vi "Basic Serial Write and Read_COM.vi"(0 "Setting":T1={"VISA resource name"="COM1", "baud rate"=57600, "data bits"=8, "parity"=0, "stop bits"=10, "flow control"=0, "Read TimeOut (ms)"=500, "Byte Read Count(999Exit)"=500, "Read End Str"=FALSE, "End String"=""} {"flow control" items=["None"=0, "XON/XOFF"=1, "RTS/CTS"=2, "DTR/DSR"=4]; "stop bits" items=["1.0"=10, "1.5"=15, "2.0"=20]; "parity" items=["None", "Odd", "Even", "Mark", "Space"]; "data bits" min=5 max=8 step=1}, 2 "string to write":string="*IDN?\n", 3 "Open":bool, 5 "write":bool=TRUE, 6 "read":bool=TRUE) -> (9 "read string":string, 10 "bytes read":u32)   [LabVIEW 2016]
doc: "The Basic Serial Read and Write example performs a Serial Port Read, a Serial Port Write, or a combination of these actions. The user selects the actions (read or write) on the front panel. If both are selected, the VI will write the data first, read data, and then close the VISA session that is opened to the port. This VI will wait until the specified number of bytes is received at the port or until a termination character is read.\n\nINSTRUCTIONS:\n1) Select the serial resource and configuration parameters (baud rate, data bits, parity, stop bits, flow control).\n2) Select the operations to be performed. \n3) Connect the serial port to your device. If no device is available, perform a loopback test by doing one of the following. Short pins 2 and 3 on a RS-232 cable or short pin 4 to pin 8 and pin 5 to pin 9 on a RS-485/422 cable. \n4) Run the VI to see the data read. (The \"read string\" will match the \"string to write\" if a loopback test was performed.)\n\nNote: The parameters set for the serial port must match the parameters of the connected instrument or device. In this example, the bytes to read parameter specifies the number of bytes that the serial port reads. If there were more bytes at the port than the number specified in bytes to read, those bytes would not be read. Also, if you specify to read more bytes than the number of bytes actually read, you might receive a timeout error message.\n\nOn the block diagram, the Configure Serial Port VI sets the configuration parameters. The front panel displays the controls used to configure the basic parameters, such as baud rate, data bits, and parity. Constants configure the other parameters the user probably does not need set. After the VISA Configure Serial Port VI opens the VISA session and configures the port, the VI passes the VISA resource name to other VIs that perform operations on that VISA resource. The VISA Write function sends a command to the serial device and the VISA Read function returns data based on the command. The VISA Close function then closes the reference to the serial device. It is important to close the reference; otherwise communication through with that port through protocols other than VISA might not be possible."
uses:
  <vilib>/Instr/_visa.llb/VISA Configure Serial Port (Instr).vi
panel:
  out "read buffer":string
  out "Tact Time":u32
  out "return count":u32
  # "On Windows/Linux, consider using the Instrument Driver Finder (Help>>Find Instrument Drivers) to search for an instrument driver for your instrument."
  # "Select the serial resource and the operations (Read, Write, or both) to be performed.  If both are selected, the VI will write the data first, read data and then close the VISA session that is opened to the port.  This VI will wait until the specified number of bytes is received at the port or until a termination character is read."
  # "For additional information select File >> VI Properties >> Documentation"
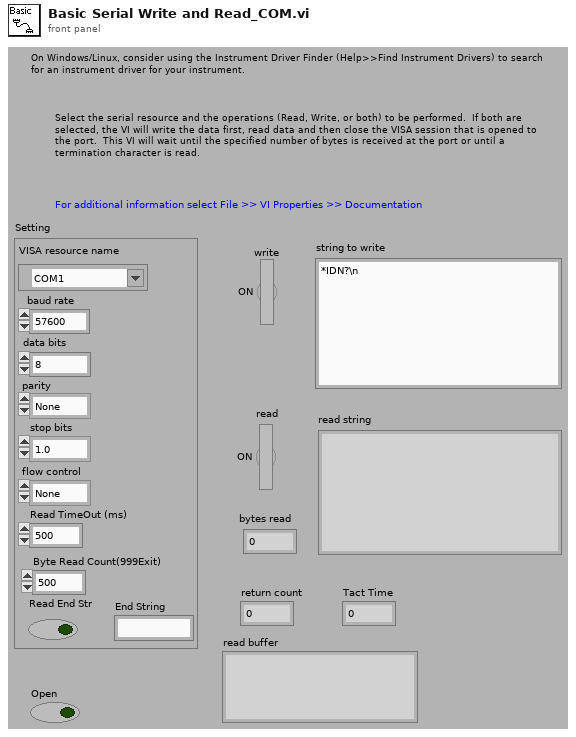
[diagram p1: front panel]
types:
  T1 = cluster{"VISA resource name":refnum<visa-resource-name>, "baud rate":u32, "data bits":u16, "parity":u16, "stop bits":u16, "flow control":u16, "Read TimeOut (ms)":u32, "Byte Read Count(999Exit)":u32, "Read End Str":bool, "End String":string}
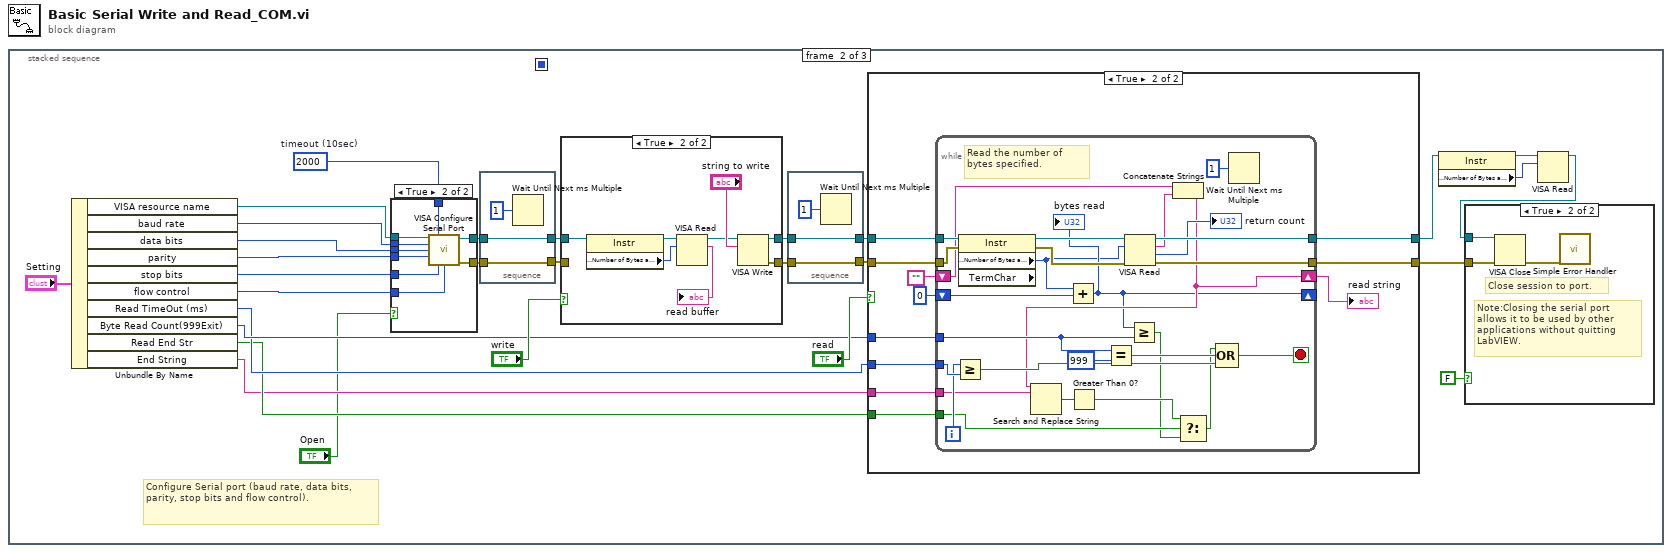
[diagram p0: block diagram]
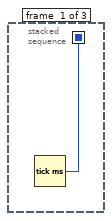
[diagram p2: hidden frame]
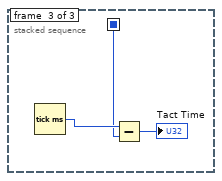
[diagram p7: hidden frame]
diagram:
  n1 = stacked-sequence {
    seq-local: [w1 _ _] -> [_ _ w101]
    frame #0 {
      n2 = Tick Count (ms)() -> (millisecond timer value=w1:u32)
    }
    frame #1 {
      w28 = u32 2000  # timeout (10sec)
      # "Configure Serial port (baud rate, data bits, parity, stop bits and flow control)."
      n3 = Unbundle By Name("Setting") -> ("VISA resource name"=w3:refnum<visa-resource-name>, "baud rate"=w25:u32, "data bits"=w24:u16, "parity"=w23:u16, "stop bits"=w22:u16, "flow control"=w21:u16, "Read TimeOut (ms)"=w19:u32, "Byte Read Count(999Exit)"=w20:u32, "Read End Str"=w18:bool, "End String"=w17:string)
      n4 = case shown="True" "Open" {
        tunnel: [_ w49] -> w9
        tunnel: [w40 w48] -> w11
        tunnel: w28 -> [_ w47]
        tunnel: w3 -> [w40 w46]
        tunnel: w25 -> [_ w45]
        tunnel: w24 -> [_ w44]
        tunnel: w23 -> [_ w43]
        tunnel: w22 -> [_ w42]
        tunnel: w21 -> [_ w41]
        frame False {
        }
        frame True {
          n5 = call-poly "VISA Configure Serial Port"("VISA resource name"=w46, "timeout (10sec)"=w47, "baud rate (9600)"=w45, "data bits (8)"=w44, "parity (0:none)"=w43, "stop bits (10: 1 bit)"=w42, "flow control (0:none)"=w41) -> ("VISA resource name out"=w48:refnum<visa-resource-name>, "error out"=w49:errorcluster)  [unwired: 2 in, 5 out]
        }
      }
      n6 = stacked-sequence {
        tunnel: w11 -> [w36]
        tunnel: [w36] -> w10
        tunnel: w9 -> [w35]
        tunnel: [w35] -> w8
        frame #0 {
          n7 = Wait Until Next ms Multiple(millisecond multiple=u32 1) -> ()  [unwired: 1 out]
        }
      }
      n8 = case shown="True" "write" {
        tunnel: [w50 w59] -> w6
        tunnel: w10 -> [w51 w57]
        tunnel: [w51 w55] -> w7
        tunnel: w8 -> [w50 _]
        frame False {
        }
        frame True {
          n9 = property class="Instr"(reference=w57) -> (reference out=w54:refnum<visa-resource-name>, "Serial Settings:Number of Bytes at Serial Port"=w53:u32)  [unwired: 1 in, 1 out]
          n10 = VISA Read(VISA resource name=w54, byte count=w53) -> (VISA resource name out=w56:refnum<visa-resource-name>, read buffer=→"read buffer":string)  [unwired: 1 in, 2 out]
          n11 = VISA Write(VISA resource name=w56, write buffer="string to write") -> (VISA resource name out=w55:refnum<visa-resource-name>, error out=w59:errorcluster)  [unwired: 1 in, 1 out]
        }
      }
      n12 = stacked-sequence {
        tunnel: w7 -> [w33]
        tunnel: [w33] -> w5
        tunnel: w6 -> [w32]
        tunnel: [w32] -> w4
        frame #0 {
          n13 = Wait Until Next ms Multiple(millisecond multiple=u32 1) -> ()  [unwired: 1 out]
        }
      }
      n14 = case shown="True" "read" {
        tunnel: w4 -> [w61 w67]
        tunnel: [w61 w65] -> w29
        tunnel: [w60 w66] -> w13
        tunnel: w5 -> [w60 w68]
        tunnel: w20 -> [_ w72]
        tunnel: w19 -> [_ w71]
        tunnel: w18 -> [_ w70]
        tunnel: w17 -> [_ w69]
        frame False {
        }
        frame True {
          n15 = while {
            tunnel: [w99] -> w65
            tunnel: [w98] -> w66
            tunnel: w68 -> [w97]
            tunnel: w67 -> [w96]
            shift-right: [w83] -> w64
            shift-left: "" -> [w93]
            shift-right: [w74] -> _
            shift-left: u32 0 -> [w91]
            tunnel: w72 -> [w88]
            tunnel: w71 -> [w85]
            tunnel: w70 -> [w80]
            tunnel: w69 -> [w77]
            i -> [w84]
            stop <- w90 stop-if-true
            # "Read the number of bytes specified."
            n16 = Greater Or Equal?(x=w84, y=w85) -> (x >= y?=w86:bool)
            n17 = property class="Instr" props=["Serial Settings:Number of Bytes at Serial Port", "TermChar"](reference=w97, error in=w96) -> (reference out=w76:refnum<visa-resource-name>, error out=w95:errorcluster, "Serial Settings:Number of Bytes at Serial Port"=w73:u32)  [unwired: 1 out]
            n18 = Add(x=w73, y=w91) -> (x+y=w74:u32)
            "bytes read" <- w74
            n19 = Equal?(x=w88, y=u32 999) -> (x = y?=w89:bool)
            n20 = VISA Read(VISA resource name=w76, byte count=w73, error in (no error)=w95) -> (VISA resource name out=w98:refnum<visa-resource-name>, read buffer=w92:string, return count=→"return count":u32, error out=w99:errorcluster)
            n21 = Greater Or Equal?(x=w74, y=w88) -> (x >= y?=w78:bool)
            n22 = Concatenate Strings(w93, w92) -> (w83:string)
            n23 = Search and Replace String(input string=w83, search string=w77) -> (number of replacements=w82:i32)  [unwired: 6 in, 3 out]
            n24 = Greater Than 0?(x=w82) -> (x > 0?=w81:bool)
            n25 = Select(t=w81, s=w80, f=w78) -> (s? t:f=w79:bool)
            n26 = Compound Arithmetic op=OR(w79, w89, w86) -> (w90:bool)
            n27 = Wait Until Next ms Multiple(millisecond multiple=u32 1) -> ()  [unwired: 1 out]
          }
          "read string" <- w64
        }
      }
      n28 = property class="Instr"(reference=w13) -> (reference out=w14:refnum<visa-resource-name>, "Serial Settings:Number of Bytes at Serial Port"=w15:u32)  [unwired: 1 in, 1 out]
      n29 = VISA Read(VISA resource name=w14, byte count=w15) -> (VISA resource name out=w12:refnum<visa-resource-name>)  [unwired: 1 in, 3 out]
      n30 = case shown="True" FALSE {
        tunnel: w29 -> [_ w39]
        tunnel: w12 -> [_ w38]
        frame False {
        }
        frame True {
          # "Note:Closing the serial port allows it to be used by other applications without quitting LabVIEW."
          # "Close session to port."
          n31 = VISA Close(VISA resource name=w38, error in (no error)=w39) -> (error out=w37:errorcluster)
          n32 = call <vilib>:"Simple Error Handler.vi"("error in (no error)"=w37) -> ()  [unwired: 1 in, 8 out]
        }
      }
    }
    frame #2 {
      n33 = Tick Count (ms)() -> (millisecond timer value=w102:u32)
      n34 = Subtract(x=w102, y=w101) -> (x-y=→"Tact Time":u32)
    }
  }
